vi "Stable.vi"(8 "Eval Period (sec)":dbl(knob)=0.5044674819294696 scale=0.0..1.0, 11 "Signal Input":bool) -> (0 "Stable":bool)   [LabVIEW 2012]
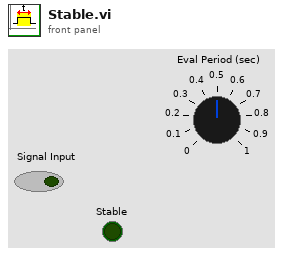
[diagram p1: front panel]
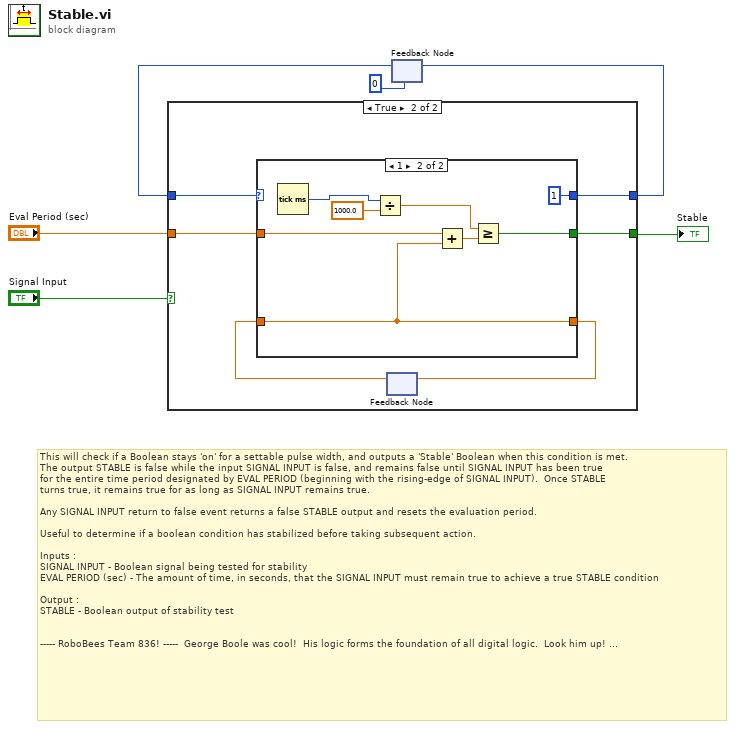
[diagram p0: block diagram]
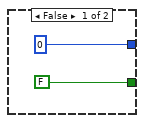
[diagram p2: hidden frame]
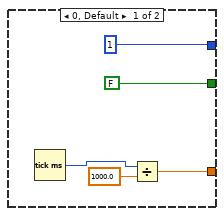
[diagram p3: hidden frame]
diagram:
  # "This will check if a Boolean stays 'on' for a settable pulse width, and outputs a 'Stable' Boolean when this condition is met.\nThe output STABLE is false while the input SIGNAL INPUT is false, and remains false until SIGNAL INPUT has been true\nfor the entire time period designated by EVAL PERIOD (beginning with the rising-edge of SIGNAL INPUT).  Once STABLE \nturns true, it remains true for as long as SIGNAL INPUT remains true.\n\nAny SIGNAL INPUT return to false event returns a false STABLE output and resets the evaluation period.\n\nUseful to determine if a boolean condition has stabilized before taking subsequent action.\n\nInputs :\nSIGNAL INPUT - Boolean signal being tested for stability\nEVAL PERIOD (sec) - The amount of time, in seconds, that the SIGNAL INPUT must remain true to achieve a true STABLE condition\n\nOutput :\nSTABLE - Boolean output of stability test\n\n\n----- RoboBees Team 836! -----  George Boole was cool!  His logic forms the foundation of all digital logic.  Look him up! ..."
  n1 = feedback #1(0) -> (w1:i32)
  n2 = case shown="True" "Signal Input" {
    tunnel: [FALSE w14] -> w6
    tunnel: "Eval Period (sec)" -> [_ w13]
    tunnel: [0 w10] -> w2
    tunnel: w1 -> [_ w9]
    frame False {
    }
    frame True {
      n3 = feedback #2() -> (w11:dbl)  [unwired: 1 in]
      n4 = case shown="1" w9 {
        tunnel: [FALSE w26] -> w14
        tunnel: w13 -> [_ w25]
        tunnel: [w15 w24] -> w12
        tunnel: w11 -> [_ w24]
        tunnel: [1 1] -> w10
        frame 0, Default {
          n5 = Tick Count (ms)() -> (millisecond timer value=w17:u32)
          n6 = Divide(x=w17, y=1000.0) -> (x/y=w15:dbl)
        }
        frame 1 {
          n7 = Tick Count (ms)() -> (millisecond timer value=w22:u32)
          n8 = Divide(x=w22, y=1000.0) -> (x/y=w20:dbl)
          n9 = Add(x=w25, y=w24) -> (x+y=w27:dbl)
          n10 = Greater Or Equal?(x=w20, y=w27) -> (x >= y?=w26:bool)
        }
      }
      n11 = feedback-in #2(w12) -> ()
    }
  }
  "Stable" <- w6
  n12 = feedback-in #1(w2) -> ()
